vi "Create.vi"(9 "Alias":string, 10 "Actor":refnum<class "Actor.lvclass">, 11 "Dev Panel in":refnum<class "Dev Panel.lvclass">) -> (3 "Dev Panel out":refnum<class "Dev Panel.lvclass">)   [LabVIEW 2021, in "Dev Panel.lvclass"]
uses:
  Dev Panel.lvclass
  Dev Panel.lvclass/Dev Panel.ctl
  Actor/Event Actor/Event Actor.lvclass
  Actor/Actor/Actor.lvclass
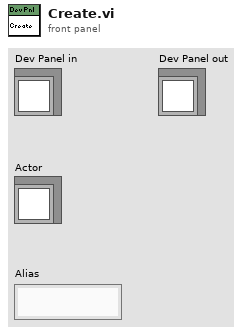
[diagram p1: front panel]
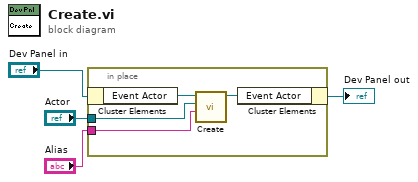
[diagram p0: block diagram]
diagram:
  n1 = in-place {
    in-place-border: "Actor" -> [w6]
    in-place-border: "Alias" -> [w5]
    n2 = in-place-cluster #1("Dev Panel in") -> ("Event Actor"=w8:refnum<class "Event Actor.lvclass">)
    n3 = call-dynamic "Create.vi"("Alias"=w5, "Actor"=w6, "Create in"=w8) -> ("Create out"=w7:refnum<class "Event Actor.lvclass">)  [unwired: 8 in]
    n4 = in-place-cluster #1("Event Actor"=w7) -> (→"Dev Panel out":refnum<class "Dev Panel.lvclass">)
  }
